vi "RBT.vi"(0 "System no.":i32=1 min=1 max=4 step=1, 5 "error in":errorcluster) -> (19 "error out":errorcluster)   [LabVIEW 2020]
doc: "GCS 3.0\n=====\n\nRBT (Reboot System)\n\nDescription\nReboots system. The system behaves in the same way as after switching on.\n\nFormat\nRBT \n\nArguments\nnone\n\nResponse\nnone\n\nNotes\nRBT must not be accepted in macros.\n\nUser command level\nUSR\n\n\nGCS 2.0\n=====\n\nReboots the controller. Controller behaves like after a cold start.\n\nC-887, F-206, M-8X0: For GCS syntax version = GCS 2.0 or higher (check with CSV?.vi. If CSV?.vi is not supported, syntax version is GCS 1.0).\n\nC-885: Reboots master only."
panel:
  # "RBT (Reboot System)\n\nReboots system. The system behaves in the same way as after switching on."
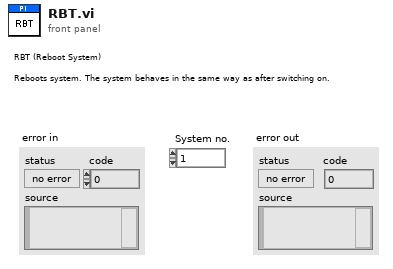
[diagram p1: front panel]
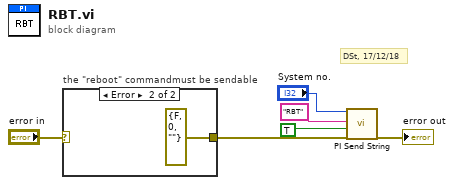
[diagram p0: block diagram]
diagram:
  # "DSt, 17/12/18"
  n1 = case "the \"reboot\" commandmust be sendable" shown="Error" "error in" {
    selector: "error in" -> [w7 _]
    tunnel: [w7 errorcluster {"status"=FALSE, "code"=0, "source"=""} ("error IO")] -> w1
    frame No Error {
    }
    frame Error {
    }
  }
  n2 = call "PI Send String.vi"("System no."="System no.", "String to send"="RBT", "Attach termination char.?"=TRUE ("Attach Linefeed?"), "error in"=w1) -> ("error out"=→"error out":errorcluster)  [unwired: 15 out]
